vi "c2f.vi"(1 "degree\nc":dbl) -> (0 "degree f":dbl)   [LabVIEW 2018]
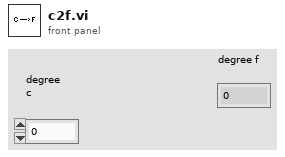
[diagram p1: front panel]
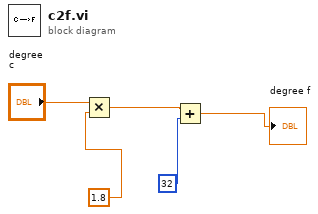
[diagram p0: block diagram]
diagram:
  n1 = Multiply(x="degree\nc", y=1.8) -> (x*y=w4:dbl)
  n2 = Add(x=w4, y=32) -> (x+y=→"degree f":dbl)
